vi "Write signal std.vi"(8 "error in (no error)":errorcluster, 10 "signal std":dbl[](array[numeric]), 11 "processingTA in":refnum<class "processingTA.lvclass">) -> (0 "error out":errorcluster, 3 "processingTA out":refnum<class "processingTA.lvclass">)   [LabVIEW 2019, in "processingTA.lvlib" / "processingTA.lvclass"]
uses:
  processingTA.lvclass
  processingTA.lvclass/processingTA.ctl
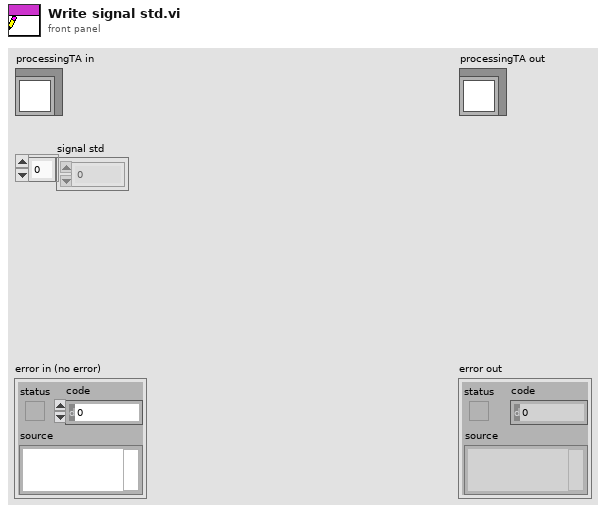
[diagram p1: front panel]
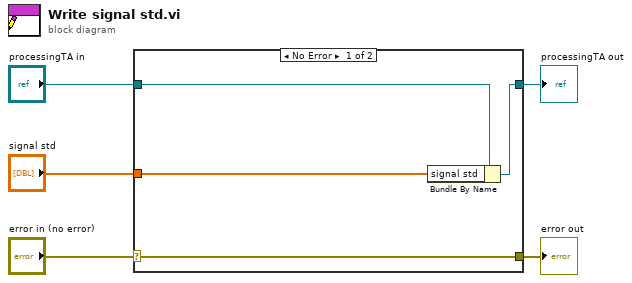
[diagram p0: block diagram]
diagram:
  n1 = case shown="No Error" "error in (no error)" {
    selector: "error in (no error)" -> [w9 w10]
    tunnel: [w9 w10] -> w4
    tunnel: [w7 w11] -> w2
    tunnel: "processingTA in" -> [w8 w11]
    tunnel: "signal std" -> [w6 _]
    frame No Error {
      n2 = Bundle By Name(cluster=w8, "signal std"=w6) -> (w7:refnum<class "processingTA.lvclass">)
    }
    frame Error {
    }
  }
  "error out" <- w4
  "processingTA out" <- w2
